vi "grSim Packet Command.vi"(7 "replace ball":bool, 8 "grSim replacement":T3={"grSim_RobotReplacement"=[{"x"=0.0, "y"=-450.0, "dir"=0.0, "yellowteam"=FALSE, "id"=0}, {"x"=0.0, "y"=-270.0, "dir"=0.0, "yellowteam"=FALSE, "id"=1}, {"x"=0.0, "y"=-90.0, "dir"=0.0, "yellowteam"=FALSE, "id"=2}, {"x"=0.0, "y"=90.0, "dir"=0.0, "yellowteam"=FALSE, "id"=3}, {"x"=0.0, "y"=270.0, "dir"=0.0, "yellowteam"=FALSE, "id"=4}, {"x"=0.0, "y"=450.0, "dir"=0.0, "yellowteam"=FALSE, "id"=5}], "grSim_BallReplacement"={"x"=0.0, "y"=0.0, "vx"=0.0, "vy"=0.0}}, 10 "Robots":T4[](array[typedef]), 11 "isteamyellow":bool=TRUE) -> (1 "Array":u8[](array[numeric]))   [LabVIEW 2018]
uses:
  Convert AI Robot to Robot Command Folder/grSim/grSim Robot Command.ctl
  grSim RobotReplacement.ctl
  grSim_BallReplacement.ctl
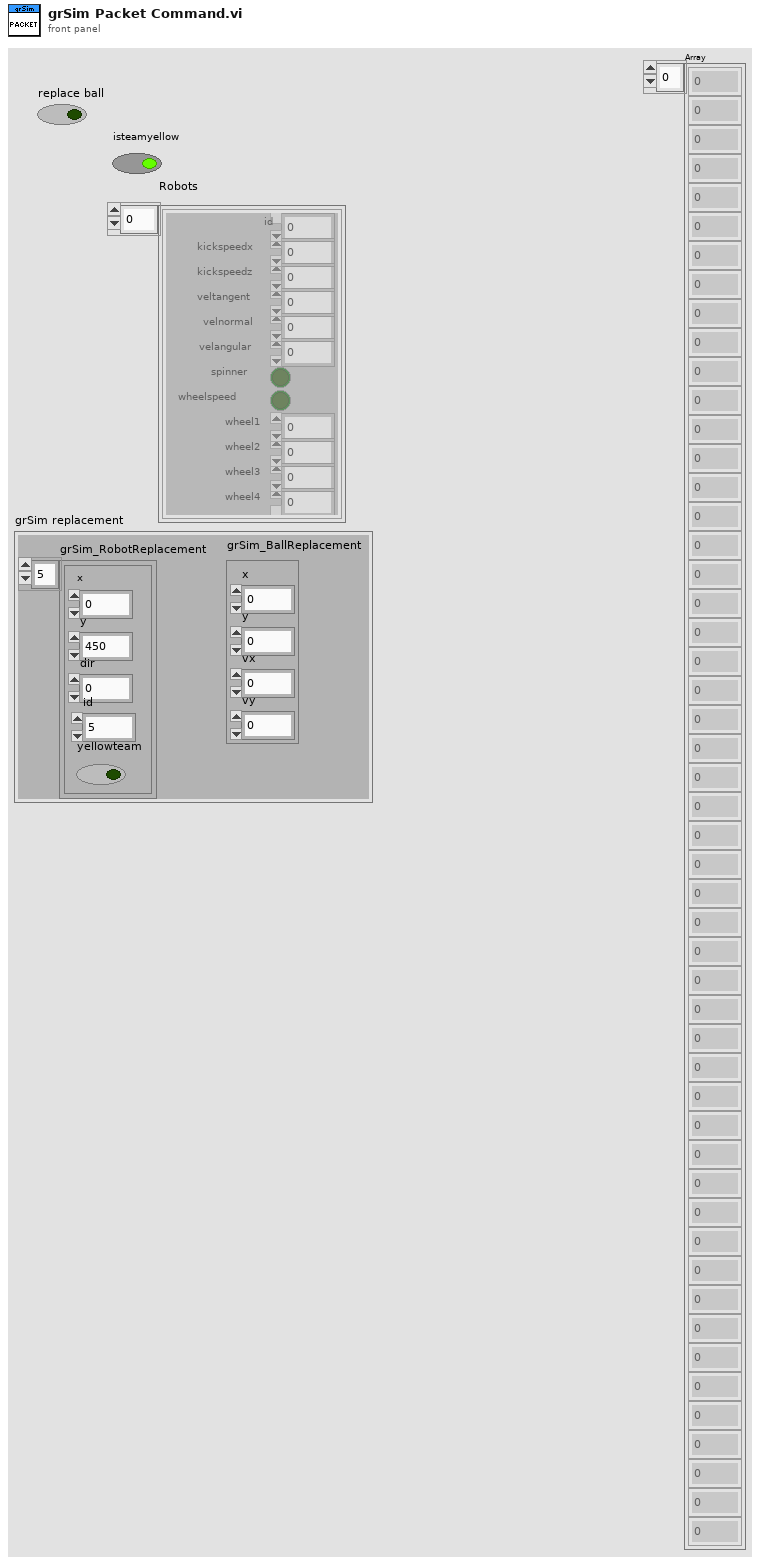
[diagram p1: front panel]
types:
  T1 = typedef "grSim RobotReplacement.ctl" = cluster{"x":dbl, "y":dbl, "dir":dbl, "yellowteam":bool, "id":u32}
  T2 = typedef "grSim_BallReplacement.ctl" = cluster{"x":dbl, "y":dbl, "vx":dbl, "vy":dbl}
  T3 = cluster{"grSim_RobotReplacement":T1[], "grSim_BallReplacement":T2}
  T4 = typedef "grSim Robot Command.ctl" = cluster{"id":u32, "kickspeedx":sgl, "kickspeedz":sgl, "veltangent":sgl, "velnormal":sgl, "velangular":sgl, "spinner":bool, "wheelspeed":bool, "wheel1":sgl, "wheel2":sgl, "wheel3":sgl, "wheel4":sgl}
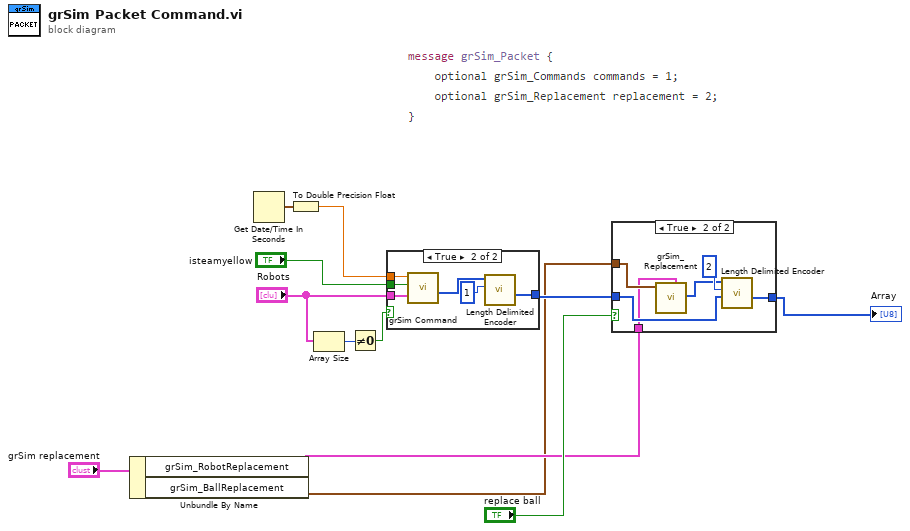
[diagram p0: block diagram]
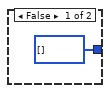
[diagram p3: hidden frame]
diagram:
  n1 = Unbundle By Name("grSim replacement") -> ("grSim_RobotReplacement"=w3:T1[], "grSim_BallReplacement"=w2:T2)
  n2 = Get Date/Time In Seconds() -> (seconds since 1Jan1904=w11:timestamp)
  n3 = To Double Precision Float(number=w11) -> (double precision float=w10:dbl)
  n4 = Array Size(array="Robots") -> (size(s)=w9:i32)
  n5 = Not Equal To 0?(x=w9) -> (x != 0?=w8:bool)
  n6 = case shown="True" w8 {
    tunnel: "isteamyellow" -> [_ w17]
    tunnel: w10 -> [_ w16]
    tunnel: [u8[] [] ("Array") w15] -> w5
    tunnel: "Robots" -> [_ w14]
    frame False {
    }
    frame True {
      n7 = call "grSim Command.vi"("Robots"=w14, "isteamyellow"=w17, "timestamp"=w16) -> ("Array"=w19:u8[])  [unwired: 8 in]
      n8 = call "Length Delimited Encoder.vi"("Key"=u32 1, "Array In 2"=w19) -> ("Array"=w15:u8[])  [unwired: 9 in]
    }
  }
  n9 = case shown="True" "replace ball" {
    tunnel: [w20 w25] -> w6
    tunnel: w3 -> [_ w21]
    tunnel: w5 -> [w20 w23]
    tunnel: w2 -> [_ w22]
    frame False {
    }
    frame True {
      n10 = call "grSim_Replacement.vi"("grSim_RobotReplacement"=w21, "grSim_BallReplacement"=w22) -> ("Array"=w24:u8[])  [unwired: 9 in]
      n11 = call "Length Delimited Encoder.vi"("Array In"=w23, "Key"=u32 2, "Array In 2"=w24) -> ("Array"=w25:u8[])  [unwired: 8 in]
    }
  }
  "Array" <- w6
